vi "Stellungen_Namen2.vi"(4 "Pumpensteuerung":dbl min=0.0 max=10.0 step=0.1, 6 "Exp.V":dbl(slide) min=0.0 max=10.0 step=1e-05 scale=0.0..10.0, 8 "Verdichterdrehzahl":dbl min=0.0 max=1500.0, 9 "zu":bool, 10 "auf":bool, 11 "RV 35 (KV)":dbl(slide) scale=0.02..0.004) -> (3 "Dynamic Data":dynamicdata(waveform) caption="Dynamischer Ausgang")   [LabVIEW 2015]
uses:
  <vilib>/express/express shared/transition.llb/Dynamic To Waveform Array.vi
  <vilib>/express/express signal manip/GetorSetDDTAttributes/Set DDT Attributes/SetT0.vi
  <vilib>/express/express shared/transition.llb/Waveform Array To Dynamic.vi
  <vilib>/express/express signal manip/GetorSetDDTAttributes/Set DDT Attributes/Set DDT Properties.xnode
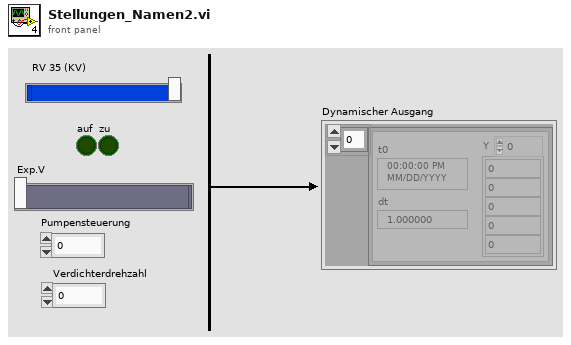
[diagram p1: front panel]
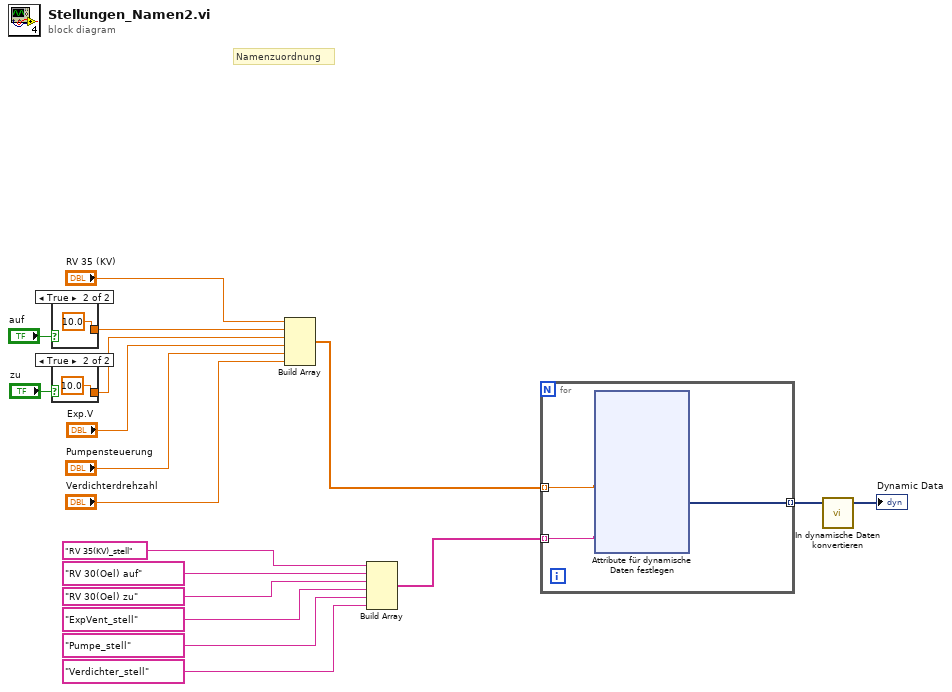
[diagram p0: block diagram]
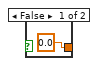
[diagram p2: hidden frame]
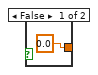
[diagram p3: hidden frame]
diagram:
  # "Namenzuordnung"
  n1 = case shown="True" "auf" {
    tunnel: [0.0 10.0] -> w15
    frame False {
    }
    frame True {
    }
  }
  n2 = case shown="True" "zu" {
    tunnel: [0.0 10.0] -> w14
    frame False {
    }
    frame True {
    }
  }
  n3 = Build Array("RV 35 (KV)", w15, w14, "Exp.V", "Pumpensteuerung", "Verdichterdrehzahl") -> (w16:dbl[])
  n4 = Build Array("RV 35(KV)_stell" ("element"), "RV 30(Oel) auf", "RV 30(Oel) zu", "ExpVent_stell", "Pumpe_stell", "Verdichter_stell") -> (w17:string[])
  n5 = for {
    tunnel: [w25] -> w12 mode=indexing
    tunnel: w17 -> [w24] mode=indexing
    tunnel: w16 -> [w23] mode=indexing
    n6 = xnode "Attribute für dynamische Daten festlegen"("Signals In"=w23, "Signal Name"=w24) -> ("Signals Out"=w25:dynamicdata)  [unwired: 2 in, 1 out]
  }
  n7 = call "In dynamische Daten konvertieren"("Array of Waveforms"=w12) -> ("Dynamic Data Type"=→"Dynamic Data":dynamicdata)  [unwired: 3 in]
